vi "error_log.vi"(9 "error":errorcluster) -> ()   [LabVIEW 2015, in "oskar_tools.lvlib"]
uses:
  Global.vi
  <vilib>/Utility/file.llb/Write Delimited Spreadsheet (string).vi
  oskar_tools.lvlib
panel:
  out "Output":path[](array[path])
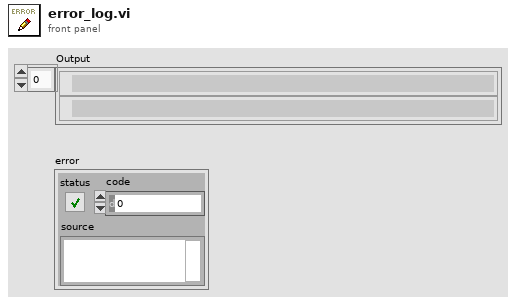
[diagram p1: front panel]
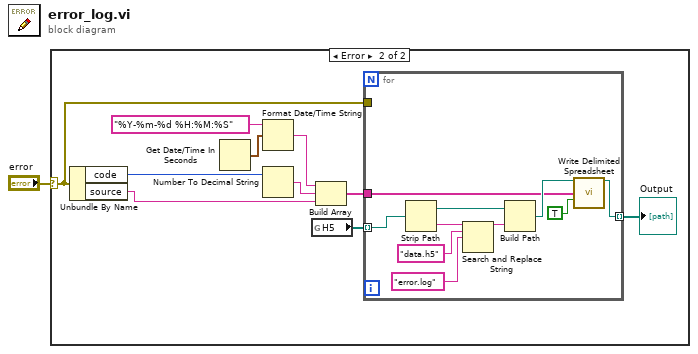
[diagram p0: block diagram]
diagram:
  n1 = case shown="Error" "error" {
    selector: "error" -> [_ w7]
    frame No Error {
    }
    frame Error {
      n2 = Unbundle By Name(w7) -> ("code"=w6:i32, "source"=w3:string)
      n3 = Get Date/Time In Seconds() -> (seconds since 1Jan1904=w8:timestamp)
      n4 = Format Date/Time String(time format string (%c)="%Y-%m-%d %H:%M:%S", seconds (now)=w8) -> (date/time string=w4:string)  [unwired: 1 in]
      n5 = Number To Decimal String(number=w6) -> (decimal integer string=w5:string)  [unwired: 1 in]
      n6 = global read "Global.vi" "H5"() -> (w11:path[])
      n7 = Build Array(w4, w5, w3) -> (w2:string[])
      n8 = for {
        tunnel: w11 -> [w21] mode=indexing
        tunnel: [w12] -> w10 mode=indexing
        tunnel: w7 -> [_]
        tunnel: w2 -> [w14]
        n9 = Strip Path(path=w21) -> (stripped path=w20:path, name=w19:string)
        n10 = Search and Replace String(input string=w19, search string="data.h5", replace string="error.log" ("replace string (\"\")")) -> (result string=w16:string)  [unwired: 5 in, 3 out]
        n11 = Build Path(base path=w20, name or relative path=w16) -> (appended path=w15:path)
        n12 = call-poly <vilib>:"Write Delimited Spreadsheet.vi"("file path (dialog if empty)"=w15, "1D data"=w14, "append to file? (F)"=TRUE ("append to file? (new file:F)")) -> ("new file path (Not A Path if cancelled)"=w12:path)  [unwired: 11 in, 1 out]
      }
      "Output" <- w10
    }
  }
